vi "Periodic Tasks.vi"(8 "error in":errorcluster) -> ()   [LabVIEW 2016]
doc: "This VI runs in parallel to other tasks. It can contain as many user-defined periodic loops as you need. These can carry out PID or other sorts of timed response."
uses:
  <vilib>/Rock Robotics/WPI/Utilities/WPI_GetSetVariantRefNum.vi
  Robot Global Data.vi
  <vilib>/Rock Robotics/Network Tables/NT Write Number.vi
  navx-mxp/labview/navX Library v2/navX Library v2.lvlib
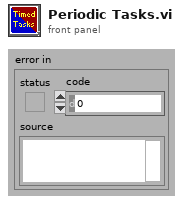
[diagram p1: front panel]
types:
  T1 = typedef "WPI_JoystickDevRef.ctl" = cluster{"Device":T2}
  T2 = typedef "WPI_JoystickDeviceEnum.ctl" = enum16{"USB 0", "USB 1", "USB 2", "USB 3", "USB 4", "USB 5"}
  T3 = typedef "WPI_RobotDriveDevRef.ctl" = cluster{"DevStatus":errorcluster, "Motors[]":T4[], "Square Inputs":bool, "Max Output":dbl}
  T4 = typedef "WPI_MotorControlDeviceRef.ctl" = cluster{"DeviceStatus":errorcluster, "Type":T5, "PWM":cluster{"PWM Channel":T6, "DeadBand":T7}, "CAN":cluster{"Device Number":u8, "SetOutput VI Ref":variant, "GetOutput VI Ref":variant, "Enable VI Ref":variant, "Disable VI Ref":variant, "Data":variant}, "Invert":bool}
  T5 = typedef "WPI_MotorControlType.ctl" = enum16{"PWM", "CAN"}
  T6 = typedef "FPGA_DIOPWMChannel.ctl" = enum8{"PWM 0", "PWM 1", "PWM 2", "PWM 3", "PWM 4", "PWM 5", "PWM 6", "PWM 7", "PWM 8", "PWM 9", "PWM MXP 0", "PWM MXP 1", "PWM MXP 2", "PWM MXP 3", "PWM MXP 4", "PWM MXP 5", "PWM MXP 6", "PWM MXP 7", "PWM MXP 8", "PWM MXP 9", "Invalid"}
  T7 = typedef "WPI_PWMDeadband.ctl" = cluster{"Name":string, "maxPositivePwm":i32, "minPositivePwm":i32, "centerPwm":i32, "maxNegativePwm":i32, "minNegativePwm":i32, "angularRange":u16}
  T8 = cluster{"JoystickDevRef":T1, "RobotDriveDevRef":T3}
  T9 = typedef "navX Library v2.lvlib/Z900_navX_DeviceTypeDef.ctl" = cluster{"Interface":cluster{"Protocol":T10, "Update Rate (4Hz-100Hz)":u8, "navX Open TypeDef":variant}, "Notify Packet":refnum<notifier>, "Loop VI Refnum":refnum<vi>, "Ready to Close Occurrence Refnum":refnum<k4>}
  T10 = typedef "navX Library v2.lvlib/Z900_navX_ProtocolTypeDef.ctl" = enum16{"SERIAL", "I2C", "SPI"}
  T11 = cluster{"Yaw":dbl, "Roll":dbl, "Pitch":dbl, "Heading":dbl, "Fused Heading":dbl}
  T12 = cluster{"Buttons[0]":bool, "Buttons[1]":bool, "Buttons[2]":bool, "Buttons[3]":bool, "Buttons[4]":bool, "Buttons[5]":bool, "Buttons[6]":bool, "Buttons[7]":bool, "Buttons[8]":bool}
  T13 = typedef "WPI_CANTalonSRX_GlobalStatus.ctl" = cluster{"Applied Throttle":dbl, "Module Enabled":bool, "CAN Error":errorcluster, "Closed Loop Error":dbl, "Forward Limit Switch Closed":bool, "Reverse Limit Switch Closed":bool, "Sensor Position":dbl, "Sensor Velocity":dbl, "Current":dbl, "Sticky Fault - Over Temp":bool, "Sticky Fault - Under Voltage":bool, "Sticky Fault - Forward Limit":bool, "Sticky Fault - Reverse Limit":bool, "Sticky Fault - Forward Soft Limit":bool, "Sticky Fault - Reverse Soft Limit":bool, "Brake is Enabled":bool, "Encoder Position":dbl, "Encoder Velocity":dbl, "Encoder Index Count":dbl, "Encoder A Pin State":bool, "Encoder B Pin State":bool, "Encoder Index Pin State":bool, "Analog In":dbl, "Analog In Velocity":dbl, "Temperature (C)":dbl, "Battery Voltage":dbl, "Control 5 Is Supported":bool, "Current Profile Slot Select":dbl, "Pos Div 8":bool, "Vel Div 4":bool, "Pulse Width Position":i32, "Pulse Width Velocity":i32, "Pulse Width Rise To Rise (us)":i32, "Pulse Width Rise To Fall (us)":i32, "Mot Prof Active Is Under Run":bool, "Mot Prof Active Has Under Run":bool, "Mot Prof Active Is Last":bool, "Mot Prof Active Velocity Only":bool, "Mot Prof Active Is Valid":bool, "Mot Prof Buffer Is Full":bool, "Mot Prof Active Profile Slot Select":i32, "Mot Prof NextID":i32, "Mot Prof Count":i32, "Mot Prof Active Velocity":dbl, "Mot Prof Active Position":dbl, "Mot Prof Output Enable":i32}
  T14 = typedef "WPI_SwitchDevRef.ctl" = cluster{"DevStatus":errorcluster, "DIO Channel":T15, "CntIndex":T16, "Normally Closed":bool}
  T15 = typedef "FPGA_DIOChannel.ctl" = enum8{"DIO 0", "DIO 1", "DIO 2", "DIO 3", "DIO 4", "DIO 5", "DIO 6", "DIO 7", "DIO 8", "DIO 9", "DIO MXP 0", "DIO MXP 1", "DIO MXP 2", "DIO MXP 3", "DIO MXP 4", "DIO MXP 5", "DIO MXP 6", "DIO MXP 7", "DIO MXP 8", "DIO MXP 9", "DIO MXP 10", "DIO MXP 11", "DIO MXP 12", "DIO MXP 13", "DIO MXP 14", "DIO MXP 15", "SPI Port CS1", "SPI Port CS2", "SPI Port CS3", "SPI Port MISO", "SPI Port MOSI", "Invalid"}
  T16 = typedef "FPGA_CounterCtrSystemIndex.ctl" = enum8{"Ctr 0", "Ctr 1", "Ctr 2", "Ctr 3", "Ctr 4", "Ctr 5", "Ctr 6", "Ctr 7", "Invalid"}
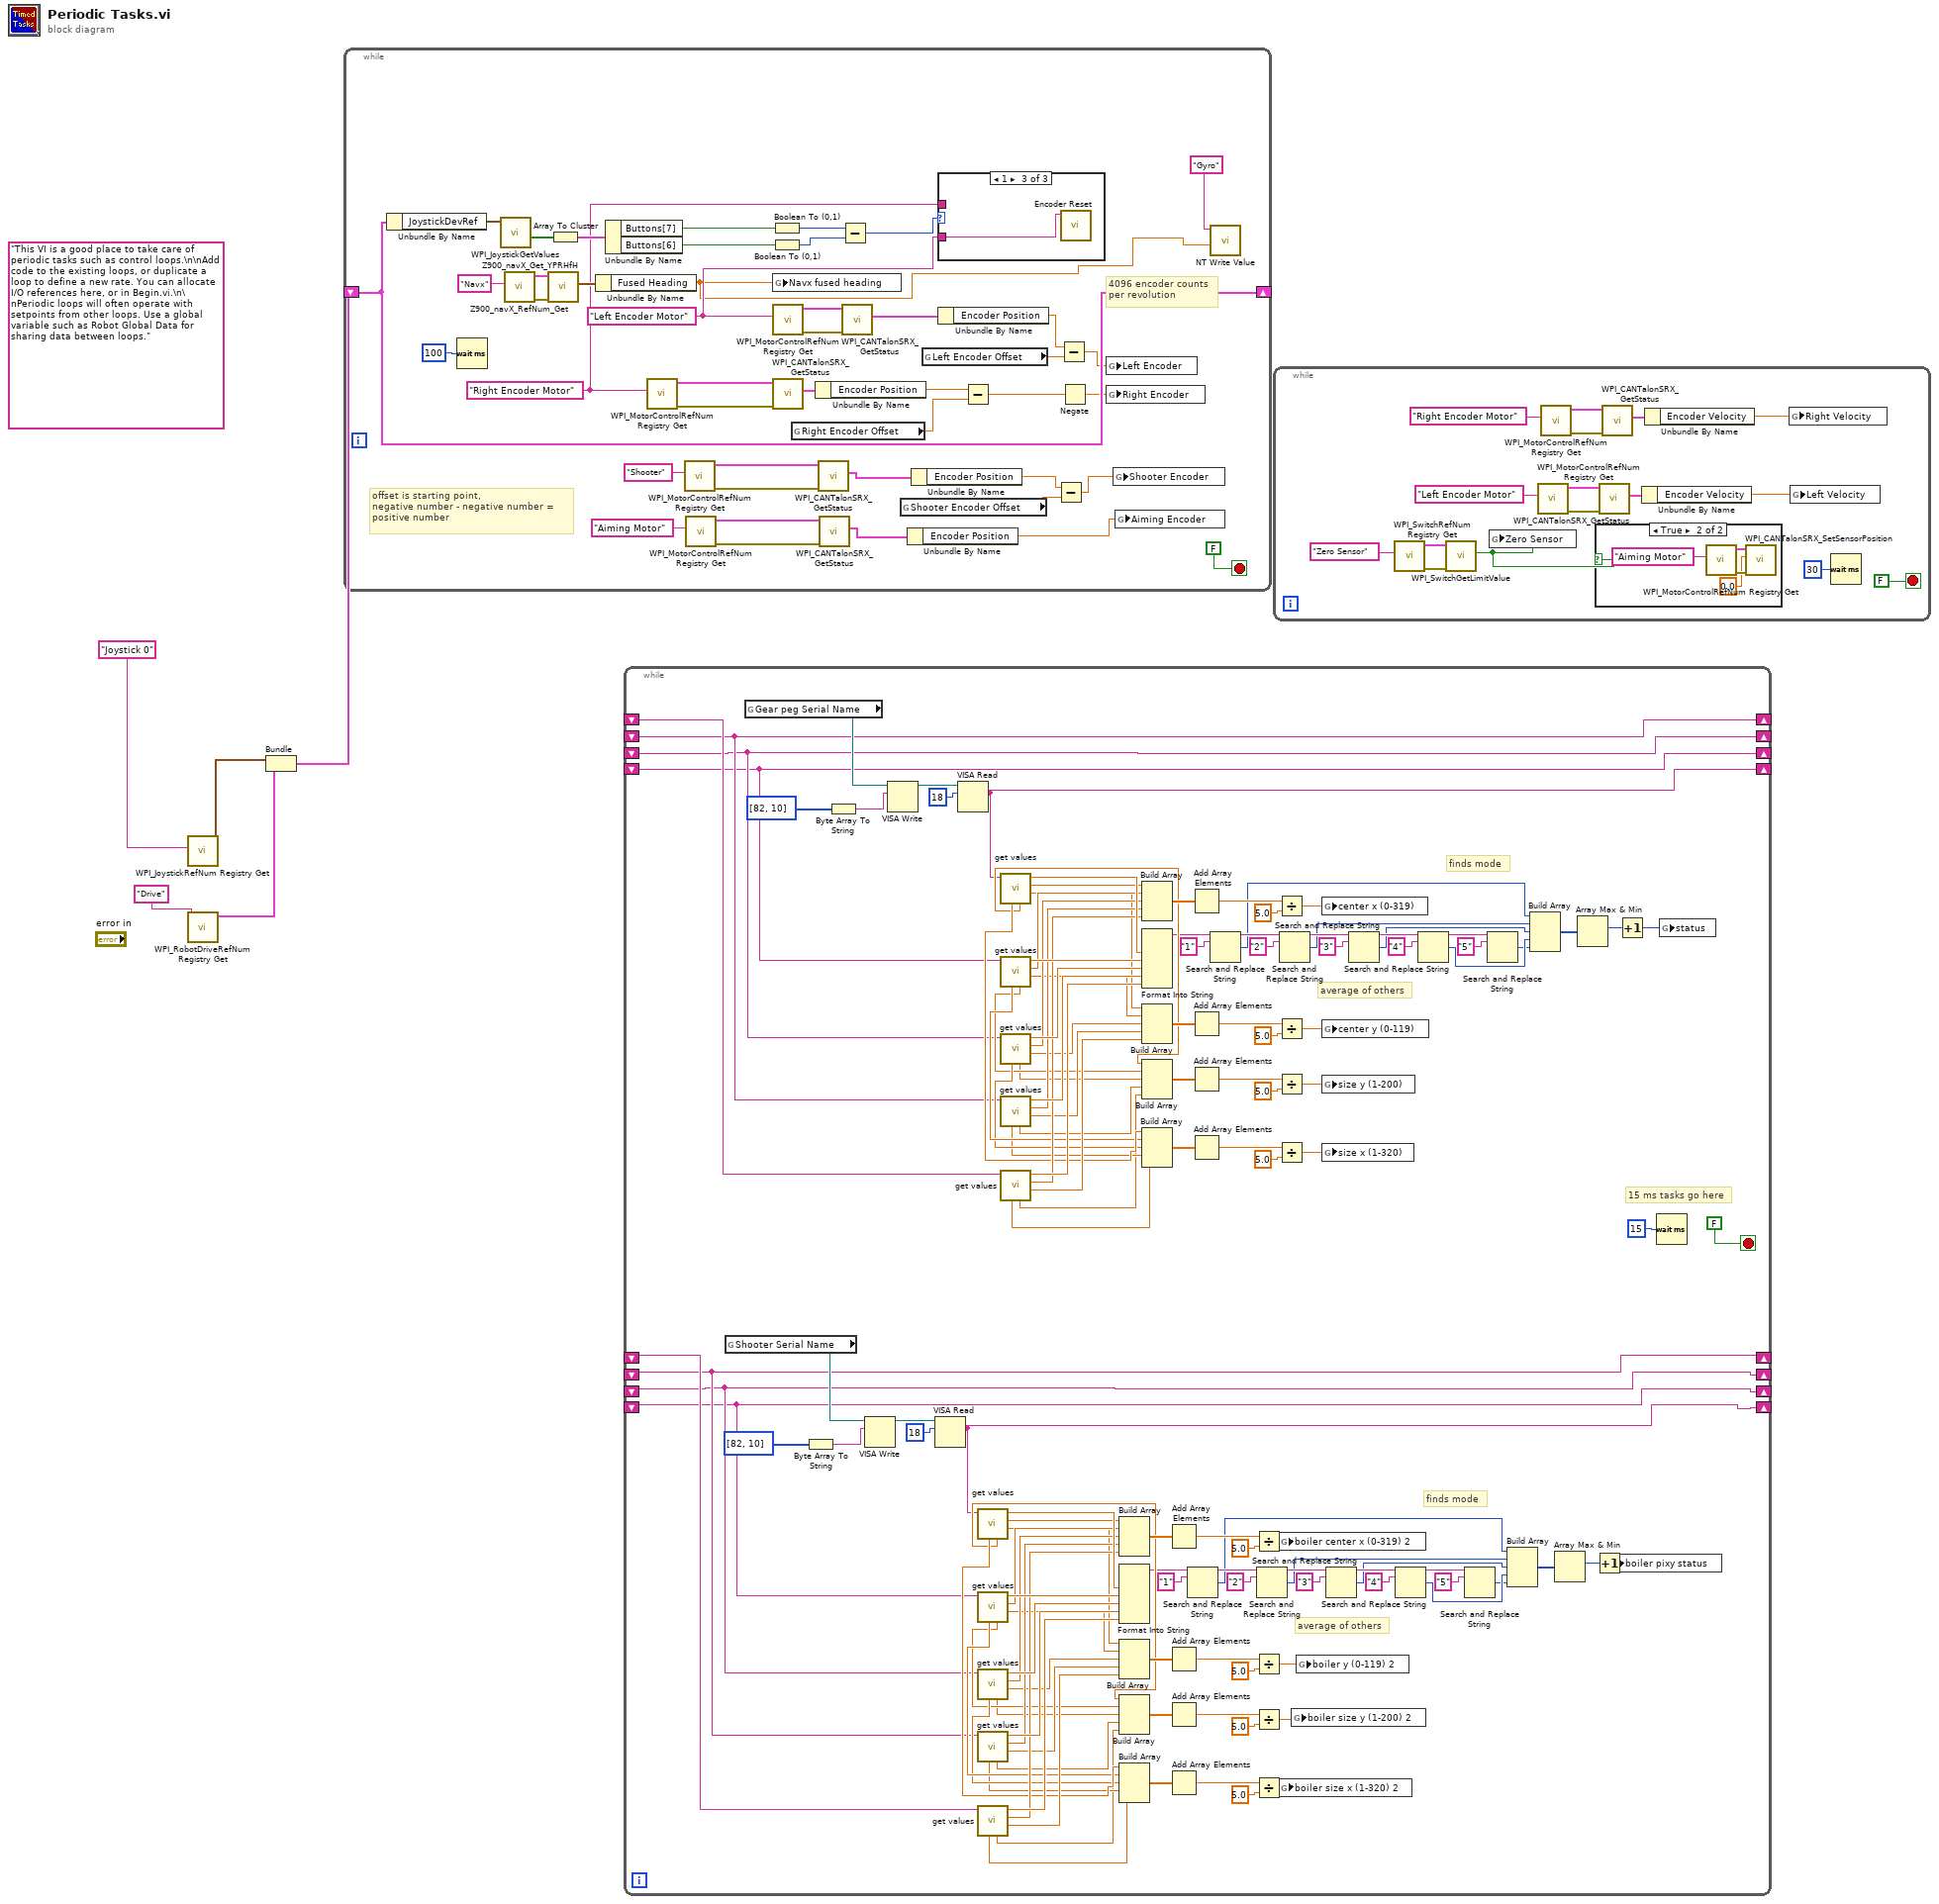
[diagram p0: block diagram]
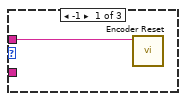
[diagram p3: hidden frame]
diagram:
  (unwired) "This VI is a good place to take care of periodic tasks such as control loops.\n\nAdd code to the existing loops, or duplicate a loop to define a new rate. You can allocate I/O references here, or in Begin.vi.\n\nPeriodic loops will often operate with setpoints from other loops. Use a global variable such as Robot Global Data for sharing data between loops."
  n1 = call <vilib>:"WPI_JoystickRefNum Registry Get.vi"("refnum name"="Joystick 0") -> ("JoystickDevRef"=w3:T1)  [unwired: 1 in, 9 out]
  n2 = call <vilib>:"WPI_RobotDriveRefNum Registry Get.vi"("refnum name"="Drive") -> ("RobotDriveDevRef"=w2:T3)  [unwired: 1 in, 9 out]
  n3 = Bundle("JoystickDevRef"=w3, "RobotDriveDevRef"=w2) -> (w1:T8)  [unwired: 1 out]
  n4 = while {
    shift-right: [w38] -> _
    shift-left: w1 -> [w38]
    stop <- FALSE stop-if-true
    w23 = "Left Encoder Motor" ("refnum name")
    w22 = "Right Encoder Motor" ("refnum name")
    # "offset is starting point,\nnegative number - negative number =\npositive number"
    # "100 ms tasks go here\n(used to be 10)"
    # "4096 encoder counts\nper revolution"
    n5 = Unbundle By Name(w38) -> ("JoystickDevRef"=w37:T1)
    n6 = Wait (ms)(milliseconds to wait=u32 100) -> ()  [unwired: 1 out]
    n7 = call <vilib>:"WPI_JoystickGetValues.vi"("JoystickDevRef"=w37) -> ("Buttons"=w36:bool[])  [unwired: 6 in, 4 out]
    n8 = call "Z900_navX_RefNum_Get.vi"("refnum name"="Navx") -> ("error out"=w42:errorcluster, "navX Device"=w43:T9)  [unwired: 9 in]
    n9 = call "Z900_navX_Get_YPRHfH.vi"("error in (no error)"=w42, "navX Device"=w43) -> ("YRPHfH"=w46:T11)  [unwired: 6 in, 3 out]
    n10 = Array To Cluster(array=w36) -> (cluster=w35:T12)
    n11 = Unbundle By Name(w46) -> ("Fused Heading"=w6:dbl)
    n12 = Unbundle By Name(w35) -> ("Buttons[7]"=w28:bool, "Buttons[6]"=w27:bool)
    n13 = call <vilib>:"WPI_MotorControlRefNum Registry Get.vi"("refnum name"=w22) -> ("error out"=w39:errorcluster, "MotorControlDevRef"=w40:T4)  [unwired: 9 in]
    n14 = call <vilib>:"WPI_MotorControlRefNum Registry Get.vi"("refnum name"="Shooter") -> ("error out"=w16:errorcluster, "MotorControlDevRef"=w15:T4)  [unwired: 9 in]
    n15 = call <vilib>:"WPI_MotorControlRefNum Registry Get.vi"("refnum name"="Aiming Motor") -> ("error out"=w17:errorcluster, "MotorControlDevRef"=w18:T4)  [unwired: 9 in]
    n16 = Boolean To (0,1)(Boolean=w28) -> (0, 1=w26:i16)
    n17 = Boolean To (0,1)(Boolean=w27) -> (0, 1=w25:i16)
    n18 = global write "Robot Global Data.vi" "Navx fused heading"(w6) -> ()
    n19 = call <vilib>:"WPI_MotorControlRefNum Registry Get.vi"("refnum name"=w23) -> ("error out"=w41:errorcluster, "MotorControlDevRef"=w34:T4)  [unwired: 9 in]
    n20 = call <vilib>:"WPI_CANTalonSRX_GetStatus.vi"("error in (no error)"=w39, "CAN Talon SRX Ref"=w40) -> ("Talon SRX Status"=w45:T13)  [unwired: 7 in, 2 out]
    n21 = global read "Robot Global Data.vi" "Right Encoder Offset"() -> (w30:dbl)
    n22 = Unbundle By Name(w45) -> ("Encoder Position"=w29:dbl)
    n23 = call <vilib>:"WPI_CANTalonSRX_GetStatus.vi"("error in (no error)"=w16, "CAN Talon SRX Ref"=w15) -> ("Talon SRX Status"=w13:T13)  [unwired: 7 in, 2 out]
    n24 = call <vilib>:"WPI_CANTalonSRX_GetStatus.vi"("error in (no error)"=w17, "CAN Talon SRX Ref"=w18) -> ("Talon SRX Status"=w12:T13)  [unwired: 7 in, 2 out]
    n25 = Subtract(x=w26, y=w25) -> (x-y=w24:i16)
    n26 = call <vilib>:"WPI_CANTalonSRX_GetStatus.vi"("error in (no error)"=w41, "CAN Talon SRX Ref"=w34) -> ("Talon SRX Status"=w44:T13)  [unwired: 7 in, 2 out]
    n27 = global read "Robot Global Data.vi" "Shooter Encoder Offset"() -> (w10:dbl)
    n28 = Unbundle By Name(w12) -> ("Encoder Position"=w8:dbl)
    n29 = Unbundle By Name(w13) -> ("Encoder Position"=w11:dbl)
    n30 = global read "Robot Global Data.vi" "Left Encoder Offset"() -> (w31:dbl)
    n31 = case shown="1" w24 {
      tunnel: w23 -> [_ _ w51]
      tunnel: w22 -> [w50 _ _]
      frame -1 {
        n32 = call "Encoder Reset.vi"("Name of Encoder"=w50) -> ()  [unwired: 11 in]
      }
      frame 0, Default {
      }
      frame 1 {
        n33 = call "Encoder Reset.vi"("Name of Encoder"=w51) -> ()  [unwired: 11 in]
      }
    }
    n34 = Unbundle By Name(w44) -> ("Encoder Position"=w33:dbl)
    n35 = Subtract(x=w29, y=w30) -> (x-y=w21:dbl)
    n36 = Subtract(x=w11, y=w10) -> (x-y=w9:dbl)
    n37 = Subtract(x=w33, y=w31) -> (x-y=w32:dbl)
    n38 = Negate(x=w21) -> (-x=w20:dbl)
    n39 = global write "Robot Global Data.vi" "Left Encoder"(w32) -> ()
    n40 = global write "Robot Global Data.vi" "Right Encoder"(w20) -> ()
    n41 = global write "Robot Global Data.vi" "Shooter Encoder"(w9) -> ()
    n42 = global write "Robot Global Data.vi" "Aiming Encoder"(w8) -> ()
    n43 = call-poly <vilib>:"NT Write Value.vi"("Numeric"=w6, "Name"="Gyro") -> ()  [unwired: 9 in, 1 out]
  }
  n44 = while {
    shift-right: [w125] -> _
    shift-left: _ -> [w121]
    shift-right: [w121] -> _
    shift-left: _ -> [w122]
    shift-right: [w123] -> _
    shift-left: _ -> [w124]
    shift-right: [w122] -> _
    shift-left: _ -> [w123]
    shift-right: [w52] -> _
    shift-left: _ -> [w53]
    shift-right: [w53] -> _
    shift-left: _ -> [w54]
    shift-right: [w55] -> _
    shift-left: _ -> [w56]
    shift-right: [w54] -> _
    shift-left: _ -> [w55]
    stop <- FALSE stop-if-true
    # "average of others"
    # "finds mode"
    # "average of others"
    # "finds mode"
    # "15 ms tasks go here"
    n45 = global read "Robot Global Data.vi" "Shooter Serial Name"() -> (w117:refnum<visa-resource-name>)
    n46 = global read "Robot Global Data.vi" "Gear peg Serial Name"() -> (w186:refnum<visa-resource-name>)
    n47 = Byte Array To String(unsigned byte array=u8[] [82, 10]) -> (string=w116:string)
    n48 = Byte Array To String(unsigned byte array=u8[] [82, 10]) -> (string=w185:string)
    n49 = VISA Write(VISA resource name=w117, write buffer=w116) -> (VISA resource name out=w119:refnum<visa-resource-name>)  [unwired: 1 in, 2 out]
    n50 = VISA Write(VISA resource name=w186, write buffer=w185) -> (VISA resource name out=w188:refnum<visa-resource-name>)  [unwired: 1 in, 2 out]
    n51 = VISA Read(VISA resource name=w119, byte count=u32 18) -> (read buffer=w52:string)  [unwired: 1 in, 3 out]
    n52 = VISA Read(VISA resource name=w188, byte count=u32 18) -> (read buffer=w125:string)  [unwired: 1 in, 3 out]
    n53 = call "get values.vi"("USB In"=w52) -> ("center y (0-119)"=w88:dbl, "center x (0-319)"=w109:dbl, "status"=w115:dbl, "size y (1-200)"=w78:dbl, "size x (1-320)"=w83:dbl)  [unwired: 6 in]
    n54 = call "get values.vi"("USB In"=w53) -> ("center y (0-119)"=w87:dbl, "center x (0-319)"=w108:dbl, "status"=w114:dbl, "size y (1-200)"=w77:dbl, "size x (1-320)"=w82:dbl)  [unwired: 6 in]
    n55 = call "get values.vi"("USB In"=w54) -> ("center y (0-119)"=w86:dbl, "center x (0-319)"=w107:dbl, "status"=w113:dbl, "size y (1-200)"=w76:dbl, "size x (1-320)"=w81:dbl)  [unwired: 6 in]
    n56 = call "get values.vi"("USB In"=w55) -> ("center y (0-119)"=w85:dbl, "center x (0-319)"=w106:dbl, "status"=w112:dbl, "size y (1-200)"=w75:dbl, "size x (1-320)"=w80:dbl)  [unwired: 6 in]
    n57 = call "get values.vi"("USB In"=w56) -> ("center y (0-119)"=w84:dbl, "center x (0-319)"=w105:dbl, "status"=w111:dbl, "size y (1-200)"=w74:dbl, "size x (1-320)"=w79:dbl)  [unwired: 6 in]
    n58 = call "get values.vi"("USB In"=w125) -> ("center y (0-119)"=w157:dbl, "center x (0-319)"=w178:dbl, "status"=w184:dbl, "size y (1-200)"=w147:dbl, "size x (1-320)"=w152:dbl)  [unwired: 6 in]
    n59 = call "get values.vi"("USB In"=w121) -> ("center y (0-119)"=w156:dbl, "center x (0-319)"=w177:dbl, "status"=w183:dbl, "size y (1-200)"=w146:dbl, "size x (1-320)"=w151:dbl)  [unwired: 6 in]
    n60 = call "get values.vi"("USB In"=w122) -> ("center y (0-119)"=w155:dbl, "center x (0-319)"=w176:dbl, "status"=w182:dbl, "size y (1-200)"=w145:dbl, "size x (1-320)"=w150:dbl)  [unwired: 6 in]
    n61 = call "get values.vi"("USB In"=w123) -> ("center y (0-119)"=w154:dbl, "center x (0-319)"=w175:dbl, "status"=w181:dbl, "size y (1-200)"=w144:dbl, "size x (1-320)"=w149:dbl)  [unwired: 6 in]
    n62 = call "get values.vi"("USB In"=w124) -> ("center y (0-119)"=w153:dbl, "center x (0-319)"=w174:dbl, "status"=w180:dbl, "size y (1-200)"=w143:dbl, "size x (1-320)"=w148:dbl)  [unwired: 6 in]
    n63 = Build Array(w109, w108, w107, w106, w105) -> (w104:dbl[])
    n64 = Format Into String(w115, w114, w113, w112, w111) -> (resulting string=w69:string)  [unwired: 3 in, 1 out]
    n65 = Build Array(w88, w87, w86, w85, w84) -> (w97:dbl[])
    n66 = Build Array(w78, w77, w76, w75, w74) -> (w89:dbl[])
    n67 = Build Array(w83, w82, w81, w80, w79) -> (w96:dbl[])
    n68 = Build Array(w178, w177, w176, w175, w174) -> (w173:dbl[])
    n69 = Format Into String(w184, w183, w182, w181, w180) -> (resulting string=w138:string)  [unwired: 3 in, 1 out]
    n70 = Build Array(w157, w156, w155, w154, w153) -> (w166:dbl[])
    n71 = Build Array(w147, w146, w145, w144, w143) -> (w158:dbl[])
    n72 = Build Array(w152, w151, w150, w149, w148) -> (w165:dbl[])
    n73 = Add Array Elements(numeric array=w104) -> (sum=w102:dbl)
    n74 = Add Array Elements(numeric array=w97) -> (sum=w99:dbl)
    n75 = Add Array Elements(numeric array=w89) -> (sum=w91:dbl)
    n76 = Add Array Elements(numeric array=w96) -> (sum=w94:dbl)
    n77 = Search and Replace String(input string=w69, search string="1") -> (result string=w68:string, number of replacements=w64:i32)  [unwired: 6 in, 2 out]
    n78 = Add Array Elements(numeric array=w173) -> (sum=w171:dbl)
    n79 = Add Array Elements(numeric array=w166) -> (sum=w168:dbl)
    n80 = Add Array Elements(numeric array=w158) -> (sum=w160:dbl)
    n81 = Add Array Elements(numeric array=w165) -> (sum=w163:dbl)
    n82 = Search and Replace String(input string=w138, search string="1") -> (result string=w137:string, number of replacements=w133:i32)  [unwired: 6 in, 2 out]
    n83 = Divide(x=w102, y=5.0) -> (x/y=w101:dbl)
    n84 = Divide(x=w99, y=5.0) -> (x/y=w100:dbl)
    n85 = Divide(x=w91, y=5.0) -> (x/y=w92:dbl)
    n86 = Divide(x=w94, y=5.0) -> (x/y=w93:dbl)
    n87 = Search and Replace String(input string=w68, search string="2") -> (result string=w67:string, number of replacements=w63:i32)  [unwired: 6 in, 2 out]
    n88 = Divide(x=w171, y=5.0) -> (x/y=w170:dbl)
    n89 = Divide(x=w168, y=5.0) -> (x/y=w169:dbl)
    n90 = Divide(x=w160, y=5.0) -> (x/y=w161:dbl)
    n91 = Divide(x=w163, y=5.0) -> (x/y=w162:dbl)
    n92 = global write "Robot Global Data.vi" "boiler center x (0-319) 2"(w101) -> ()
    n93 = global write "Robot Global Data.vi" "boiler size x (1-320) 2"(w93) -> ()
    n94 = Search and Replace String(input string=w137, search string="2") -> (result string=w136:string, number of replacements=w132:i32)  [unwired: 6 in, 2 out]
    n95 = global write "Robot Global Data.vi" "boiler size y (1-200) 2"(w92) -> ()
    n96 = global write "Robot Global Data.vi" "boiler y (0-119) 2"(w100) -> ()
    n97 = global write "Robot Global Data.vi" "center x (0-319)"(w170) -> ()
    n98 = global write "Robot Global Data.vi" "center y (0-119)"(w169) -> ()
    n99 = global write "Robot Global Data.vi" "size y (1-200)"(w161) -> ()
    n100 = global write "Robot Global Data.vi" "size x (1-320)"(w162) -> ()
    n101 = Search and Replace String(input string=w67, search string="3") -> (result string=w66:string, number of replacements=w62:i32)  [unwired: 6 in, 2 out]
    n102 = Search and Replace String(input string=w136, search string="3") -> (result string=w135:string, number of replacements=w131:i32)  [unwired: 6 in, 2 out]
    n103 = Search and Replace String(input string=w66, search string="4") -> (result string=w65:string, number of replacements=w61:i32)  [unwired: 6 in, 2 out]
    n104 = Search and Replace String(input string=w135, search string="4") -> (result string=w134:string, number of replacements=w130:i32)  [unwired: 6 in, 2 out]
    n105 = Search and Replace String(input string=w65, search string="5") -> (number of replacements=w60:i32)  [unwired: 6 in, 3 out]
    n106 = Search and Replace String(input string=w134, search string="5") -> (number of replacements=w129:i32)  [unwired: 6 in, 3 out]
    n107 = Build Array(w64, w63, w62, w61, w60) -> (w59:i32[])
    n108 = Build Array(w133, w132, w131, w130, w129) -> (w128:i32[])
    n109 = Array Max & Min(array=w59) -> (max index (indices)=w58:i32)  [unwired: 3 out]
    n110 = Array Max & Min(array=w128) -> (max index (indices)=w127:i32)  [unwired: 3 out]
    n111 = Increment(x=w58) -> (x+1=w57:i32)
    n112 = global write "Robot Global Data.vi" "boiler pixy status"(w57) -> ()
    n113 = Increment(x=w127) -> (x+1=w126:i32)
    n114 = Wait (ms)(milliseconds to wait=u32 15) -> ()  [unwired: 1 out]
    n115 = global write "Robot Global Data.vi" "status"(w126) -> ()
  }
  n116 = while {
    stop <- FALSE stop-if-true
    n117 = call <vilib>:"WPI_SwitchRefNum Registry Get.vi"("refnum name"="Zero Sensor") -> ("error out"=w194:errorcluster, "SwitchDevRef"=w193:T14)  [unwired: 9 in]
    n118 = call <vilib>:"WPI_SwitchGetLimitValue.vi"("error in (no error)"=w194, "SwitchDevRef"=w193) -> ("Switch Pressed"=w192:bool)  [unwired: 7 in, 2 out]
    n119 = global write "Robot Global Data.vi" "Zero Sensor"(w192) -> ()
    n120 = call <vilib>:"WPI_MotorControlRefNum Registry Get.vi"("refnum name"="Left Encoder Motor") -> ("error out"=w198:errorcluster, "MotorControlDevRef"=w197:T4)  [unwired: 9 in]
    n121 = call <vilib>:"WPI_MotorControlRefNum Registry Get.vi"("refnum name"="Right Encoder Motor") -> ("error out"=w203:errorcluster, "MotorControlDevRef"=w204:T4)  [unwired: 9 in]
    n122 = case shown="True" w192 {
      frame False {
      }
      frame True {
        n123 = call <vilib>:"WPI_MotorControlRefNum Registry Get.vi"("refnum name"="Aiming Motor") -> ("error out"=w210:errorcluster, "MotorControlDevRef"=w209:T4)  [unwired: 9 in]
        n124 = call <vilib>:"WPI_CANTalonSRX_SetSensorPosition.vi"("error in (no error)"=w210, "New Sensor Position"=0.0, "CAN Talon SRX Ref"=w209) -> ()  [unwired: 7 in, 2 out]
      }
    }
    n125 = call <vilib>:"WPI_CANTalonSRX_GetStatus.vi"("error in (no error)"=w198, "CAN Talon SRX Ref"=w197) -> ("Talon SRX Status"=w196:T13)  [unwired: 7 in, 2 out]
    n126 = call <vilib>:"WPI_CANTalonSRX_GetStatus.vi"("error in (no error)"=w203, "CAN Talon SRX Ref"=w204) -> ("Talon SRX Status"=w205:T13)  [unwired: 7 in, 2 out]
    n127 = Unbundle By Name(w196) -> ("Encoder Velocity"=w200:dbl)
    n128 = Unbundle By Name(w205) -> ("Encoder Velocity"=w201:dbl)
    n129 = global write "Robot Global Data.vi" "Right Velocity"(w201) -> ()
    n130 = global write "Robot Global Data.vi" "Left Velocity"(w200) -> ()
    n131 = Wait (ms)(milliseconds to wait=u32 30) -> ()  [unwired: 1 out]
  }
